vi "Auton Master.vi"() -> ()   [LabVIEW 2016]
uses:
  Auton - Boiler Gear States.ctl
  Auton - Far Gear States.ctl
  Auton - Center Gear States.ctl
  Auton - Center Gear No Vision States.ctl
  Auton - Center Gear-Basline States.ctl
  Auton - Boiler Shoot States.ctl
  Auton - Center Shoot States.ctl
  Auton - Boiler Gear Shoot States.ctl
  Auton - Center Gear Shoot States.ctl
  Auton - Drive Forward States.ctl
  <vilib>/Rock Robotics/Network Tables/NT Read Number.vi
  Robot Values.vi
  LED Send Global.vi
  Auton - Drive Forward and Turn States.ctl
panel:
  out "Auton Select":T1(ring)
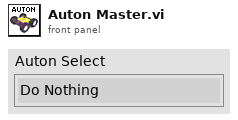
[diagram p1: front panel]
types:
  T1 = enum16{"Do Nothing", "Boiler Gear", "Far Gear", "Center Gear", "Center Gear No Vision", "Center Gear Baseline Left", "Boiler Shoot", "Center Shoot", "Boiler Gear Shoot", "Center Gear Shoot", "Boiler Bucket Shoot", "Far Gear Bucket Cross", "Drive Forward"}
  T2 = enum16{"Do Nothing", "Boiler Gear", "Far Gear", "Center Gear", "Center Gear Baseline Right", "Center Gear Baseline Left", "Boiler Shoot", "Center Shoot", "Boiler Gear Shoot", "Center Gear Shoot", "Boiler Bucket Shoot", "Far Gear Bucket Cross"}
  T3 = typedef "Robot Values.ctl" = cluster{"Robot Drive":cluster{"Left Motor Power":dbl, "Right Motor Power":dbl, "Left Encoder Value":dbl, "Right Encoder Value":dbl, "High Gear?":bool, "PTO?":bool}, "Sensors":cluster{"Gyro Angle":u16, "Recalibrate Gyro":bool, "Reset Gyro":bool, "Ultrasonic":dbl}, "Shooter":cluster{"Prep Wheels":bool, "Shoot":bool, "Left Shooter Wheel Speed":dbl, "Wheels Moving":bool, "Shooter Prepped":bool, "Shooter RPS SP":dbl, "Shooting?":bool, "Left Shooter Wheel Power":dbl, "Right Shooter Wheel Power":dbl, "Acquisition Conveyor Power":dbl, "Hopper Beater Bar Power":dbl, "Filtered Left Shooter Speed":dbl, "Acquisition Motor Power":dbl, "Joystick Add":dbl, "D-Pad Add":dbl, "Shooter Use PID?":bool}, "Robot States":cluster{"Drive mode":string, "Alliance":T4, "Position":T5}, "Gear":cluster{"Ejection Active":bool}}
  T4 = typedef "WPI_DriverStationAllianceInfo.ctl" = enum16{"Red", "Blue", "Invalid"}
  T5 = typedef "WPI_DriverStationPositionInfo.ctl" = enum16{"1", "2", "3"}
  T6 = typedef "Auton - Boiler Gear States.ctl" = enum16{"Stop", "Reset Encoders", "Drive Forward", "Face Airship Gyro", "Reset Encoders Again", "Drive Forward to Peg", "Turn to Mount Peg", "Mount Peg", "Eject Gear", "Back Away", "Reset Encoders Again Again"}
  T7 = typedef "Auton - Far Gear States.ctl" = enum16{"Stop", "Reset Encoders", "Drive Forward", "Face Airship Gyro", "Reset Encoders Again", "Drive Forward to Peg", "Turn to Mount Peg", "Reset Encoders Again Again", "Mount Peg", "Eject Gear", "Back Away"}
  T8 = typedef "Auton - Center Gear States.ctl" = enum16{"Stop", "Wait For Target", "Reset Encoders", "Drive Forward", "Turn  To Mount Peg", "Reset Encoders Again", "Mount Peg", "Eject Gear", "Back Away"}
  T9 = typedef "Auton - Drive Forward and Turn States.ctl" = enum16{"Stop", "Drive Forward", "Turn Left"}
  T10 = typedef "Auton - Center Gear No Vision States.ctl" = enum16{"Stop", "Reset Encoders", "Drive to Peg", "Eject Gear", "Back Away"}
  T11 = typedef "Auton - Center Gear-Basline States.ctl" = enum16{"Stop", "Reset Encoders", "Drive Forward", "Eject Gear", "Back Away", "Turn Away from Airship", "Reset Encoders Again", "Cross Baseline"}
  T12 = typedef "Auton - Boiler Shoot States.ctl" = enum16{"Stop", "Reset Encoders", "Drive Forward", "Turn toward boiler", "Reset Encoders Again", "Drive to boiler", "Shoot", "Back from Boiler", "Turn to Zero", "Reset Encoders Again Again", "Cross Baseline"}
  T13 = typedef "Auton - Center Shoot States.ctl" = enum16{"Stop", "Reset Encoders", "Drive Off Wall", "Turn to continue", "Reset Encoders Again", "Move toward Boiler", "Turn to Boiler", "Reset Encoders 3", "Move to Boiler", "Shoot"}
  T14 = typedef "Auton - Boiler Gear Shoot States.ctl" = enum16{"Stop", "Reset Encoders", "Drive Forward", "Face Airship Gyro", "Reset Encoders Again", "Go to Target", "Turn to Mount Gear", "Reset Encoders Mount", "Mount Gear", "Eject Gear", "Back Away from Gear", "Turn to Boiler", "Reset Encoders Boiler", "Move to Boiler", "Shoot", "Back Away from Boiler"}
  T15 = typedef "Auton - Center Gear Shoot States.ctl" = enum16{"Stop", "Reset Encoders", "Go to Target", "Turn to Mount Gear", "Reset Encoders Mount", "Mount Gear", "Eject Gear", "Back Away from Gear", "Turn Toward Boiler", "Reset Encoder Toward Boiler", "Drive Toward Boiler", "Turn to Boiler", "Reset Encoders Boiler", "Move to Boiler", "Shoot"}
  T16 = typedef "Auton - Drive Forward States.ctl" = enum16{"Stop", "Reset Encoders", "Drive Forward"}
  T17 = typedef "LED Send Global.ctl" = cluster{"Underglow States":cluster{"RED":bool, "BLUE":bool}, "Hopper States":cluster{"No Shooter Power":bool, "1 RED":bool, "2 RED":bool, "3 RED":bool, "1 YEL 3 RED":bool, "2 YEL 3 RED":bool, "3 YEL 3 RED":bool, "1 GRN 3 YEL 3 RED":bool, "2 GRN 3 YEL 3 RED":bool, "3 GRN 3 YEL 3 RED":bool, "All GRN":bool, "Shooter w/Agitator":bool}, "License Plate States":cluster{"Auton States":cluster{"Do Nothing":bool, "Gear":bool, "Gear & Baseline":bool, "Gear & Shooter":bool, "Shooter":bool, "Shooter & Ball Dump":bool}, "Drive Train":cluster{"High Gear":bool, "Low Gear":bool}}, "Misc":cluster{"Pit/Demo":bool}, "Lights":cluster{"Underglow":string, "License Plate":string, "Hopper":string}}
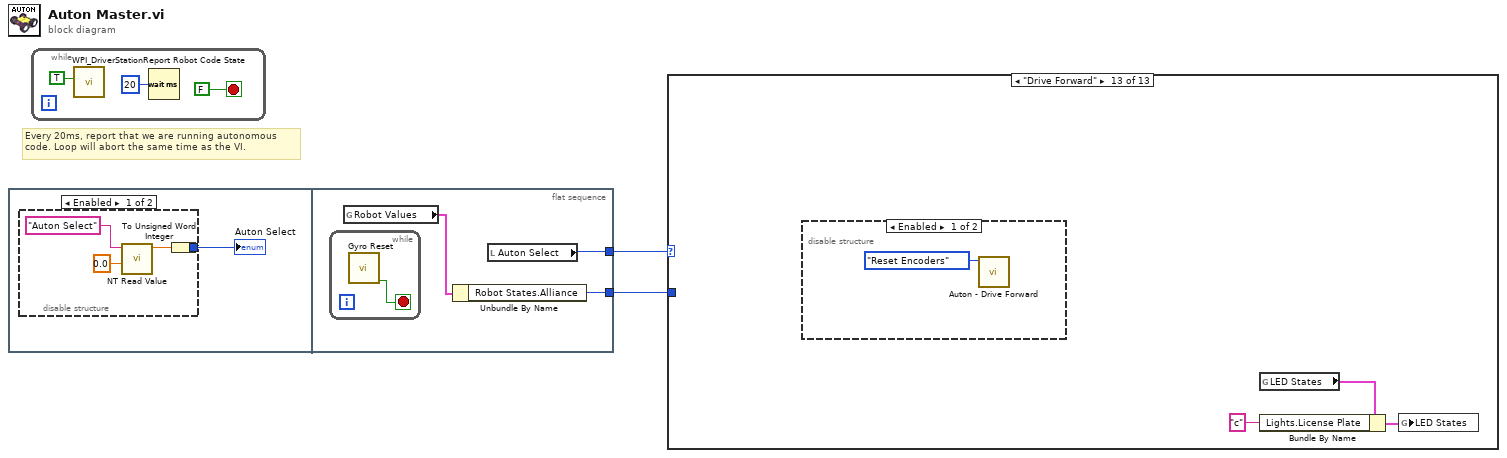
[diagram p0: block diagram]
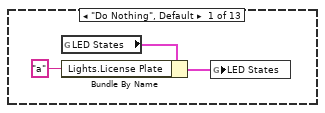
[diagram p2: hidden frame]
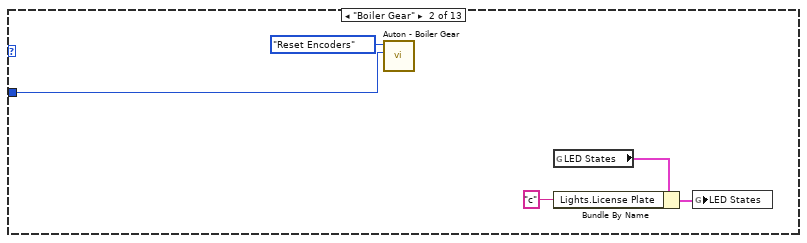
[diagram p3: hidden frame]
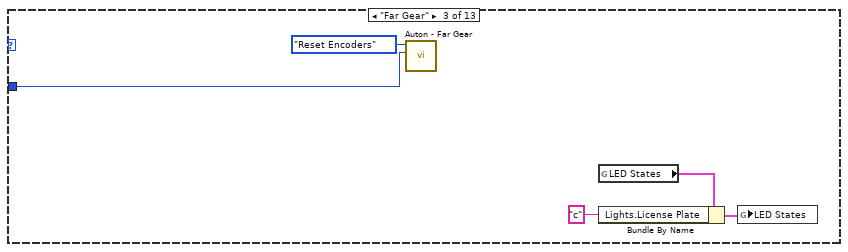
[diagram p4: hidden frame]
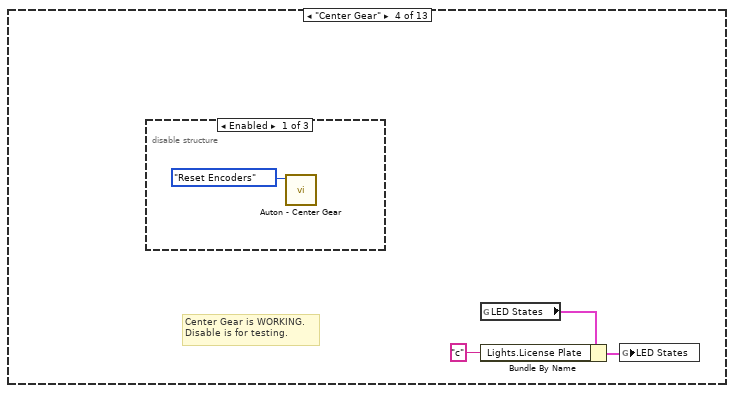
[diagram p5: hidden frame]
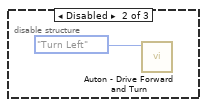
[diagram p6: hidden frame]
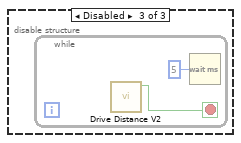
[diagram p7: hidden frame]
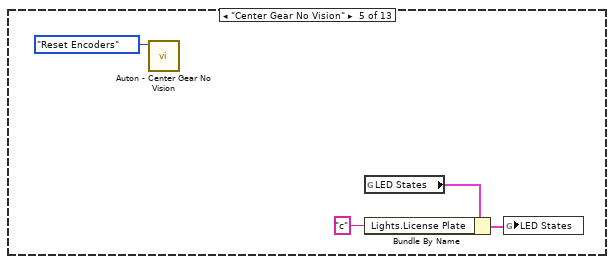
[diagram p8: hidden frame]
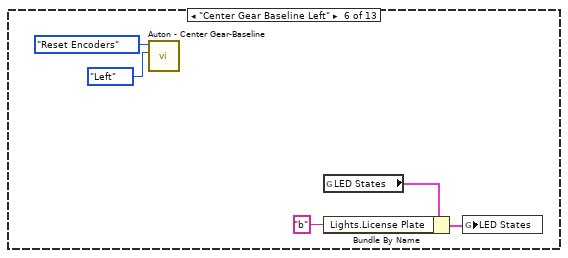
[diagram p9: hidden frame]
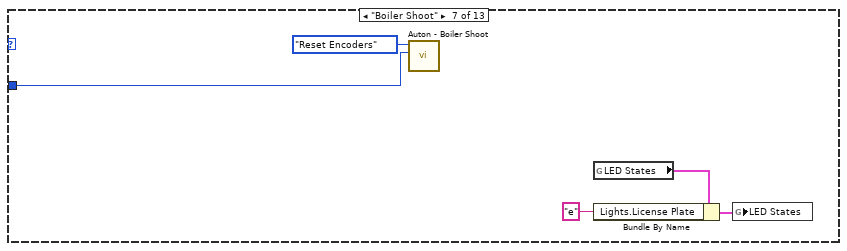
[diagram p10: hidden frame]
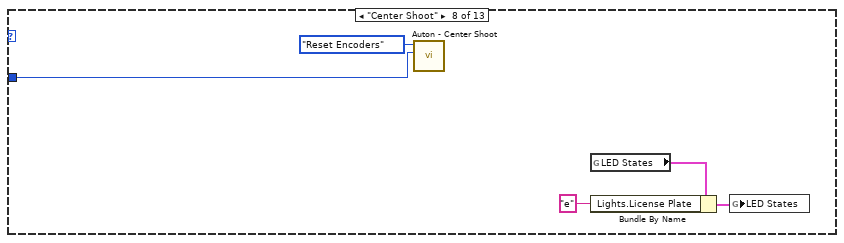
[diagram p11: hidden frame]
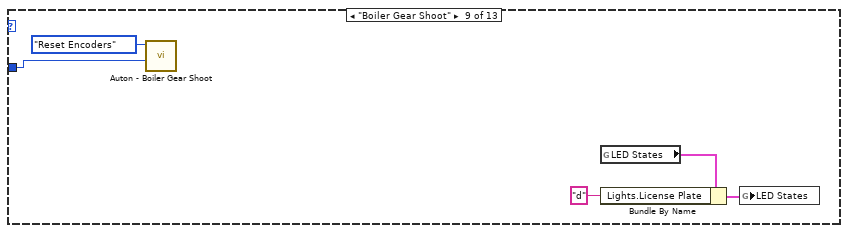
[diagram p12: hidden frame]
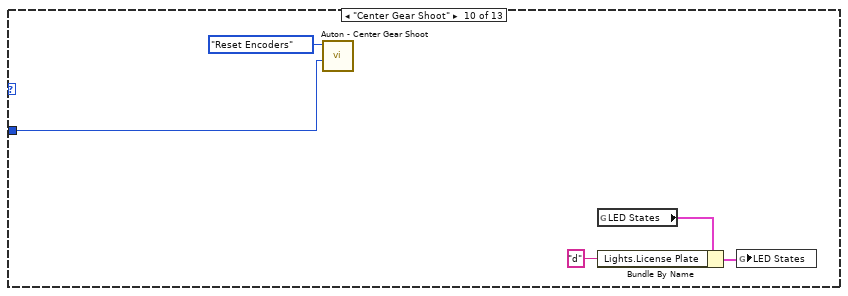
[diagram p13: hidden frame]
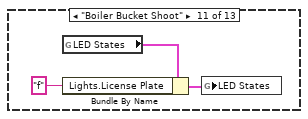
[diagram p14: hidden frame]
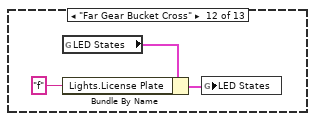
[diagram p15: hidden frame]
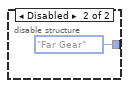
[diagram p17: hidden frame]
diagram:
  # "Every 20ms, report that we are running autonomous\ncode. Loop will abort the same time as the VI."
  n1 = flat-sequence {
    tunnel: [w11] -> w2
    tunnel: [w10] -> w1
    frame #0 {
      n2 = disable-structure shown="Enabled" {
        disable-tunnel: [w4 T2."Far Gear" ("Auton Select")] -> w3
        frame Enabled {
          n3 = call-poly <vilib>:"NT Read Value.vi"("Default Value"=0.0, "Name"="Auton Select") -> ("Numeric"=w7:dbl)  [unwired: 8 in, 1 out]
          n4 = To Unsigned Word Integer(number=w7) -> (unsigned 16bit integer=w4:u16)
        }
        frame Disabled {
        }
      }
      "Auton Select" <- w3
    }
    frame #1 {
      n5 = while {
        stop <- w12 stop-if-true
        n6 = call "Gyro Reset.vi"() -> ("Done"=w12:bool)  [unwired: 11 in]
      }
      n7 = global read "Robot Values.vi" "Robot Values"() -> (w9:T3)
      n8 = Unbundle By Name(w9) -> ("Robot States.Alliance"=w10:T4)
      n9 = local read "Auton Select"() -> (w11:T1)
    }
  }
  n10 = while {
    stop <- FALSE stop-if-true
    n11 = call <vilib>:"WPI_DriverStationReport Robot Code State.vi"("Autonomous"=TRUE) -> ()  [unwired: 10 in, 1 out]
    n12 = Wait (ms)(milliseconds to wait=u32 20) -> ()  [unwired: 1 out]
  }
  n13 = case shown="\"Drive Forward\"" w2 {
    tunnel: w1 -> [_ w22 w28 _ _ _ w49 w54 w59 w60 _ _ _]
    frame "Do Nothing", Default {
      n14 = global read "LED Send Global.vi" "LED States"() -> (w16:T17)
      n15 = Bundle By Name(cluster=w16, "Lights.License Plate"="a") -> (w17:T17)
      n16 = global write "LED Send Global.vi" "LED States"(w17) -> ()
    }
    frame "Boiler Gear" {
      n17 = call "Auton - Boiler Gear.vi"("Alliance"=w22, "Auton States"=Auton_-_Boiler_Gear_States."Reset Encoders") -> ()  [unwired: 10 in]
      n18 = global read "LED Send Global.vi" "LED States"() -> (w19:T17)
      n19 = Bundle By Name(cluster=w19, "Lights.License Plate"="c") -> (w20:T17)
      n20 = global write "LED Send Global.vi" "LED States"(w20) -> ()
    }
    frame "Far Gear" {
      n21 = call "Auton - Far Gear.vi"("Alliance"=w28, "Auton States"=Auton_-_Far_Gear_States."Reset Encoders") -> ()  [unwired: 10 in]
      n22 = global read "LED Send Global.vi" "LED States"() -> (w24:T17)
      n23 = Bundle By Name(cluster=w24, "Lights.License Plate"="c") -> (w25:T17)
      n24 = global write "LED Send Global.vi" "LED States"(w25) -> ()
    }
    frame "Center Gear" {
      # "Center Gear is WORKING.\nDisable is for testing."
      n25 = disable-structure shown="Enabled" {
        frame Enabled {
          n26 = call "Auton - Center Gear.vi"("Auton States"=Auton_-_Center_Gear_States."Reset Encoders") -> ()  [unwired: 11 in]
        }
        frame Disabled {
          n27 = call "Auton - Drive Forward and Turn.vi"("Auton States"=Auton_-_Drive_Forward_and_Turn_States."Turn Left") -> ()  [unwired: 11 in]
        }
        frame Disabled {
          n28 = while {
            stop <- w35 stop-if-true
            n29 = call "Drive Distance V2.vi"() -> ("Done?"=w35:bool)  [unwired: 11 in]
            n30 = Wait (ms)(milliseconds to wait=u32 5) -> ()  [unwired: 1 out]
          }
        }
      }
      n31 = global read "LED Send Global.vi" "LED States"() -> (w29:T17)
      n32 = Bundle By Name(cluster=w29, "Lights.License Plate"="c") -> (w30:T17)
      n33 = global write "LED Send Global.vi" "LED States"(w30) -> ()
    }
    frame "Center Gear No Vision" {
      n34 = call "Auton - Center Gear No Vision.vi"("Auton States"=Auton_-_Center_Gear_No_Vision_States."Reset Encoders") -> ()  [unwired: 11 in]
      n35 = global read "LED Send Global.vi" "LED States"() -> (w37:T17)
      n36 = Bundle By Name(cluster=w37, "Lights.License Plate"="c") -> (w38:T17)
      n37 = global write "LED Send Global.vi" "LED States"(w38) -> ()
    }
    frame "Center Gear Baseline Left" {
      n38 = call "Auton - Center Gear-Baseline.vi"("Baseline Direction"=enum16{"Right", "Left"}."Left", "Auton States"=Auton_-_Center_Gear-Basline_States."Reset Encoders") -> ()  [unwired: 10 in]
      n39 = global read "LED Send Global.vi" "LED States"() -> (w40:T17)
      n40 = Bundle By Name(cluster=w40, "Lights.License Plate"="b") -> (w41:T17)
      n41 = global write "LED Send Global.vi" "LED States"(w41) -> ()
    }
    frame "Boiler Shoot" {
      n42 = call "Auton - Boiler Shoot.vi"("Alliance"=w49, "Auton States"=Auton_-_Boiler_Shoot_States."Reset Encoders") -> ()  [unwired: 10 in]
      n43 = global read "LED Send Global.vi" "LED States"() -> (w45:T17)
      n44 = Bundle By Name(cluster=w45, "Lights.License Plate"="e") -> (w46:T17)
      n45 = global write "LED Send Global.vi" "LED States"(w46) -> ()
    }
    frame "Center Shoot" {
      n46 = call "Auton - Center Shoot.vi"("Alliance"=w54, "Auton States"=Auton_-_Center_Shoot_States."Reset Encoders") -> ()  [unwired: 10 in]
      n47 = global read "LED Send Global.vi" "LED States"() -> (w50:T17)
      n48 = Bundle By Name(cluster=w50, "Lights.License Plate"="e") -> (w51:T17)
      n49 = global write "LED Send Global.vi" "LED States"(w51) -> ()
    }
    frame "Boiler Gear Shoot" {
      n50 = call "Auton - Boiler Gear Shoot.vi"("Alliance"=w59, "Auton States"=Auton_-_Boiler_Gear_Shoot_States."Reset Encoders") -> ()  [unwired: 10 in]
      n51 = global read "LED Send Global.vi" "LED States"() -> (w55:T17)
      n52 = Bundle By Name(cluster=w55, "Lights.License Plate"="d") -> (w56:T17)
      n53 = global write "LED Send Global.vi" "LED States"(w56) -> ()
    }
    frame "Center Gear Shoot" {
      n54 = call "Auton - Center Gear Shoot.vi"("Alliance"=w60, "Auton States"=Auton_-_Center_Gear_Shoot_States."Reset Encoders") -> ()  [unwired: 10 in]
      n55 = global read "LED Send Global.vi" "LED States"() -> (w62:T17)
      n56 = Bundle By Name(cluster=w62, "Lights.License Plate"="d") -> (w63:T17)
      n57 = global write "LED Send Global.vi" "LED States"(w63) -> ()
    }
    frame "Boiler Bucket Shoot" {
      n58 = global read "LED Send Global.vi" "LED States"() -> (w65:T17)
      n59 = Bundle By Name(cluster=w65, "Lights.License Plate"="f") -> (w66:T17)
      n60 = global write "LED Send Global.vi" "LED States"(w66) -> ()
    }
    frame "Far Gear Bucket Cross" {
      n61 = global read "LED Send Global.vi" "LED States"() -> (w68:T17)
      n62 = Bundle By Name(cluster=w68, "Lights.License Plate"="f") -> (w69:T17)
      n63 = global write "LED Send Global.vi" "LED States"(w69) -> ()
    }
    frame "Drive Forward" {
      n64 = disable-structure shown="Enabled" {
        frame Enabled {
          n65 = call "Auton - Drive Forward.vi"("Auton States"=Auton_-_Drive_Forward_States."Reset Encoders") -> ()  [unwired: 11 in]
        }
        frame Disabled {
        }
      }
      n66 = global read "LED Send Global.vi" "LED States"() -> (w71:T17)
      n67 = Bundle By Name(cluster=w71, "Lights.License Plate"="c") -> (w72:T17)
      n68 = global write "LED Send Global.vi" "LED States"(w72) -> ()
    }
  }
